vi "Convert to JPEG String and Compress.vi"(10 "Image":T1(plugin-control)=refnum) -> (2 "JPEG Image String":string)   [LabVIEW 2025]
uses:
  <vilib>/vision/NI_Vision_Development_Module.lvlib
panel:
  out "Y Resolution":i32
  out "X Resolution":i32
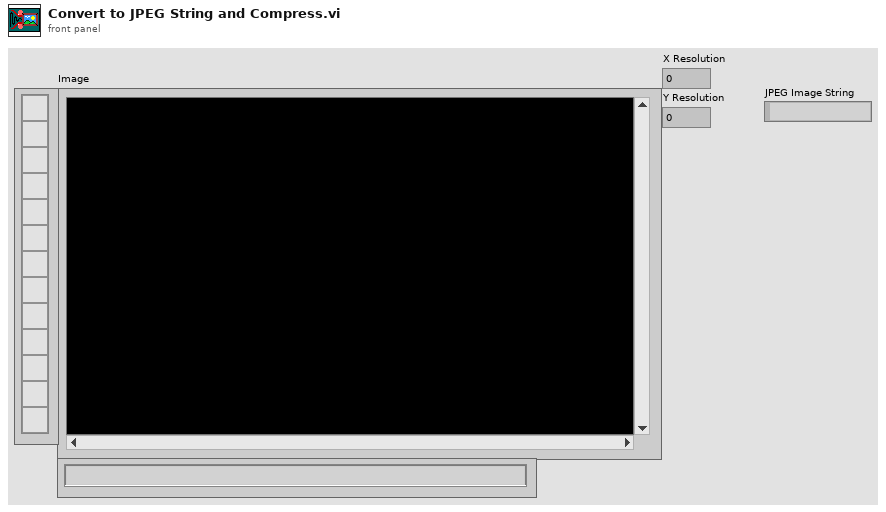
[diagram p1: front panel]
types:
  T1 = typedef "IMAQ Image.ctl" = refnum<image>
  T2 = typedef "Image Type" = u32
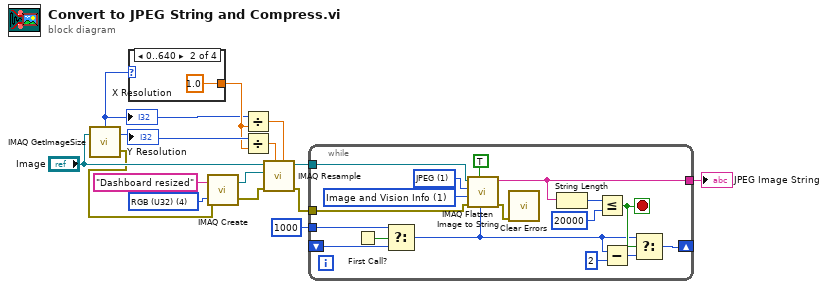
[diagram p0: block diagram]
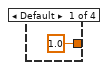
[diagram p2: hidden frame]
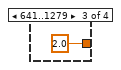
[diagram p3: hidden frame]
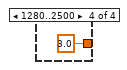
[diagram p4: hidden frame]
diagram:
  w14 = T2 4 items=["Grayscale (U8)", "Grayscale (I16)", "Grayscale (SGL)", "Complex (CSG)", "RGB (U32)", "HSL (U32)", "RGB (U64)", "Grayscale (U16)"] ("Image Type")
  n1 = call "IMAQ GetImageSize"("Image"="Image") -> ("Y Resolution"=w6:i32, "X Resolution"=w2:i32, "error out"=w1:errorcluster)  [unwired: 3 in]
  "X Resolution" <- w2
  "Y Resolution" <- w6
  n2 = case shown="0..640" w2 {
    tunnel: [1.0 ("y") 1.0 ("y") 2.0 ("y") 3.0 ("y")] -> w3
    frame Default {
    }
    frame 0..640 {
    }
    frame 641..1279 {
    }
    frame 1280..2500 {
    }
  }
  n3 = call "IMAQ Create"("Image Name"="Dashboard resized" ("string"), "Image Type"=w14, "error in (no error)"=w1) -> ("New Image"=w11:T1, "error out"=w8:errorcluster)  [unwired: 1 in, 1 out]
  n4 = Divide(x=w2, y=w3) -> (x/y=w4:sgl)
  n5 = Divide(x=w6, y=w3) -> (x/y=w5:sgl)
  n6 = call "IMAQ Resample"("X Resolution"=w4, "Y Resolution"=w5, "error in (no error)"=w8, "Image Dst"=w11, "Image Src"="Image") -> ("error out"=w13:errorcluster, "Image Dst Out"=w12:T1)  [unwired: 5 in]
  n7 = while {
    tunnel: w13 -> [w34]
    tunnel: w12 -> [w32]
    tunnel: [w30] -> w10
    shift-right: [w24] -> _
    shift-left: _ -> [w21]
    tunnel: 1000 -> [w23]
    stop <- w27 stop-if-true
    w35 = 1 items=["Image", "Image and Vision Info", "Reference to Image"] ("Type of Flatten (Image and Vision Info)")
    w36 = 1 items=["None", "JPEG", "PACKED BINARY"] ("Compression (None)")
    n8 = First Call?() -> (First Call?: T/F=w22:bool)
    n9 = Select(t=w23, s=w22, f=w21) -> (s? t:f=w20:i32)
    n10 = call "IMAQ Flatten Image to String"("Quality (750)"=w20, "Flatten with Process-Unique Name (F)"=TRUE, "error in (no error)"=w34, "Type of Flatten (Image and Vision Info)"=w35, "Compression (None)"=w36, "Image"=w32) -> ("error out"=w33:errorcluster, "Data String"=w30:string)  [unwired: 4 in]
    n11 = call <vilib>:"Clear Errors.vi"("error in (no error)"=w33) -> ()  [unwired: 5 in, 2 out]
    n12 = String Length(string=w30) -> (length=w28:i32)
    n13 = Less Or Equal?(x=w28, y=20000) -> (x <= y?=w27:bool)
    n14 = Subtract(x=w20, y=2) -> (x-y=w26:i32)
    n15 = Select(t=w20, s=w27, f=w26) -> (s? t:f=w24:i32)
  }
  "JPEG Image String" <- w10
